vi "AddToScene.vi"(8 "error in (no error)":errorcluster, 10 "sceneRoot in":refnum<class "SceneRoot.lvclass">, 11 "class data in":refnum<class "BoundingBox.lvclass">) -> (0 "error out":errorcluster, 3 "class data out":refnum<class "BoundingBox.lvclass">)   [LabVIEW 2010, in "Labricks.lvlib" / "BoundingBox.lvclass"]
doc: "Adds the scene object to the given scene."
uses:
  BoundingBox.lvclass
  RenderBase/SceneRoot_class/SceneRoot.lvclass
  BoundingBox.lvclass/BoundingBox.ctl
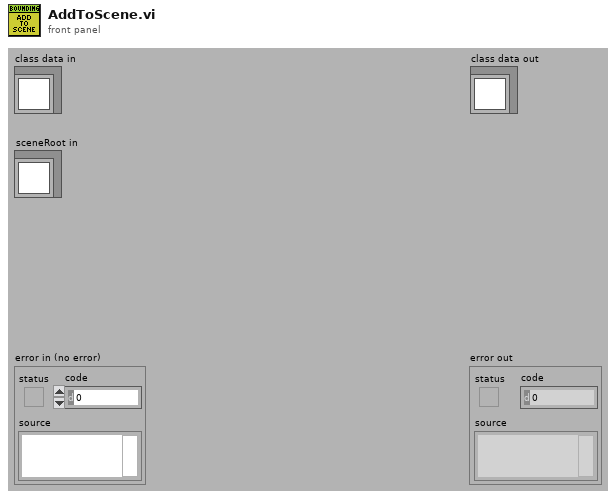
[diagram p1: front panel]
types:
  T1 = cluster{"X":sgl, "Y":sgl, "Width":sgl, "Height":sgl}
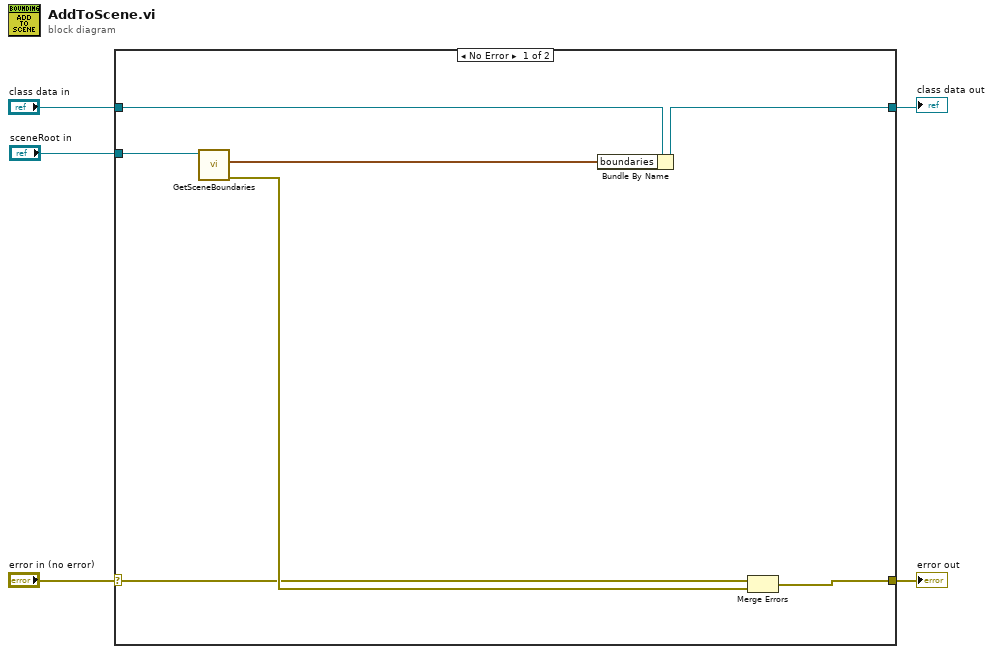
[diagram p0: block diagram]
diagram:
  n1 = case shown="No Error" "error in (no error)" {
    selector: "error in (no error)" -> [w6 w14]
    tunnel: [w7 w14] -> w4
    tunnel: "class data in" -> [w12 w13]
    tunnel: [w11 w13] -> w2
    tunnel: "sceneRoot in" -> [w10 _]
    frame No Error {
      n2 = call "GetSceneBoundaries.vi"("class data in"=w10) -> ("error out"=w8:errorcluster, "boundaries out"=w9:T1)  [unwired: 8 in, 1 out]
      n3 = Bundle By Name(cluster=w12, "boundaries"=w9) -> (w11:refnum<class "BoundingBox.lvclass">)
      n4 = Merge Errors(w6, w8) -> (w7:errorcluster)
    }
    frame Error {
    }
  }
  "error out" <- w4
  "class data out" <- w2
